vi "DIALOG_Method Selection.vi"(7 "Action":T6, 8 "Error In":errorcluster, 9 "User VI Ref":refnum<vi>, 10 "Affected Items":T4, 11 "Methods for Tree In":T5(array[cluster])=[{"Label"="Divider", "Tag"="0,6,MCListbox (strict),Divider,Divider", "Property Type"=enum."Divider", "Indent"=0, "Can Read?"=FALSE, "Can Write?"=FALSE, "Is Read?"=FALSE, "Is Write?"=FALSE, "Inactive Parent?"=FALSE, "Unwired?"=FALSE}, {"Label"="Class Operator", "Tag"="1,2,MCListbox (strict),6327405,Class Operator", "Property Type"=enum."Base", "Indent"=0, "Can Read?"=FALSE, "Can Write?"=FALSE, "Is Read?"=FALSE, "Is Write?"=FALSE, "Inactive Parent?"=TRUE, "Unwired?"=FALSE}, {"Label"="Call", "Tag"="1,2,MCListbox (strict),6327405,Class Operator:Call", "Property Type"=enum."Scripting", "Indent"=1, "Can Read?"=FALSE, "Can Write?"=FALSE, "Is Read?"=FALSE, "Is Write?"=FALSE, "Inactive Parent?"=FALSE, "Unwired?"=FALSE}, {"Label"="Traverse", "Tag"="2,2,MCListbox (strict),6327406,Class Operator:Traverse", "Property Type"=enum."Scripting", "Indent"=1, "Can Read?"=FALSE, "Can Write?"=FALSE, "Is Read?"=FALSE, "Is Write?"=FALSE, "Inactive Parent?"=FALSE, "Unwired?"=FALSE}, {"Label"="Delete", "Tag"="3,2,MCListbox (strict),6327400,Delete", "Property Type"=enum."Scripting", "Indent"=0, "Can Read?"=FALSE, "Can Write?"=FALSE, "Is Read?"=FALSE, "Is Write?"=FALSE, "Inactive Parent?"=FALSE, "Unwired?"=FALSE}, {"Label"="Get Property", "Tag"="4,3,MCListbox (strict),6327408,Get Property", "Property Type"=enum."Private", "Indent"=0, "Can Read?"=FALSE, "Can Write?"=FALSE, "Is Read?"=FALSE, "Is Write?"=FALSE, "Inactive Parent?"=FALSE, "Unwired?"=FALSE}, {"Label"="Get Property Call Data", "Tag"="5,3,MCListbox (strict),6327409,Get Property Call Data", "Property Type"=enum."Private", "Indent"=0, "Can Read?"=FALSE, "Can Write?"=FALSE, "Is Read?"=FALSE, "Is Write?"=FALSE, "Inactive Parent?"=FALSE, "Unwired?"=FALSE}, {"Label"="NI Security", "Tag"="6,3,MCListbox (strict),632740b,NI Security", "Property Type"=enum."Base", "Indent"=0, "Can Read?"=FALSE, "Can Write?"=FALSE, "Is Read?"=FALSE, "Is Write?"=FALSE, "Inactive Parent?"=TRUE, "Unwired?"=FALSE}, {"Label"="Get Access Control List", "Tag"="6,3,MCListbox (strict),632740b,NI Security:Get Access Control List", "Property Type"=enum."Private", "Indent"=1, "Can Read?"=FALSE, "Can Write?"=FALSE, "Is Read?"=FALSE, "Is Write?"=FALSE, "Inactive Parent?"=FALSE, "Unwired?"=FALSE}, {"Label"="Remove Access Control List", "Tag"="7,3,MCListbox (strict),632740c,NI Security:Remove Access Control List", "Property Type"=enum."Private", "Indent"=1, "Can Read?"=FALSE, "Can Write?"=FALSE, "Is Read?"=FALSE, "Is Write?"=FALSE, "Inactive Parent?"=FALSE, "Unwired?"=FALSE}, {"Label"="Set Access Control List", "Tag"="8,3,MCListbox (strict),632740a,NI Security:Set Access Control List", "Property Type"=enum."Private", "Indent"=1, "Can Read?"=FALSE, "Can Write?"=FALSE, "Is Read?"=FALSE, "Is Write?"=FALSE, "Inactive Parent?"=FALSE, "Unwired?"=FALSE}, {"Label"="Set HeapDocMod For Object", "Tag"="9,3,MCListbox (strict),632740d,Set HeapDocMod For Object", "Property Type"=enum."Private", "Indent"=0, "Can Read?"=FALSE, "Can Write?"=FALSE, "Is Read?"=FALSE, "Is Write?"=FALSE, "Inactive Parent?"=FALSE, "Unwired?"=FALSE}, {"Label"="Set Property", "Tag"="10,3,MCListbox (strict),6327407,Set Property", "Property Type"=enum."Private", "Indent"=0, "Can Read?"=FALSE, "Can Write?"=FALSE, "Is Read?"=FALSE, "Is Write?"=FALSE, "Inactive Parent?"=FALSE, "Unwired?"=FALSE}, {"Label"="Tag", "Tag"="11,2,MCListbox (strict),6327403,Tag", "Property Type"=enum."Base", "Indent"=0, "Can Read?"=FALSE, "Can Write?"=FALSE, "Is Read?"=FALSE, "Is Write?"=FALSE, "Inactive Parent?"=TRUE, "Unwired?"=FALSE}, {"Label"="Get Tag", "Tag"="11,2,MCListbox (strict),6327403,Tag:Get Tag", "Property Type"=enum."Scripting", "Indent"=1, "Can Read?"=FALSE, "Can Write?"=FALSE, "Is Read?"=FALSE, "Is Write?"=FALSE, "Inactive Parent?"=FALSE, "Unwired?"=FALSE}, {"Label"="Remove Tag", "Tag"="12,2,MCListbox (strict),6327402,Tag:Remove Tag", "Property Type"=enum."Scripting", "Indent"=1, "Can Read?"=FALSE, "Can Write?"=FALSE, "Is Read?"=FALSE, "Is Write?"=FALSE, "Inactive Parent?"=FALSE, "Unwired?"=FALSE}, {"Label"="Set Tag", "Tag"="13,2,MCListbox (strict),6327401,Tag:Set Tag", "Property Type"=enum."Scripting", "Indent"=1, "Can Read?"=FALSE, "Can Write?"=FALSE, "Is Read?"=FALSE, "Is Write?"=FALSE, "Inactive Parent?"=FALSE, "Unwired?"=FALSE}, {"Label"="Set Tag Persistence", "Tag"="14,2,MCListbox (strict),6327404,Tag:Set Tag Persistence", "Property Type"=enum."Scripting", "Indent"=1, "Can Read?"=FALSE, "Can Write?"=FALSE, "Is Read?"=FALSE, "Is Write?"=FALSE, "Inactive Parent?"=FALSE, "Unwired?"=FALSE}, {"Label"="Divider", "Tag"="15,6,MCListbox (strict),Divider,Divider", "Property Type"=enum."Divider", "Indent"=0, "Can Read?"=FALSE, "Can Write?"=FALSE, "Is Read?"=FALSE, "Is Write?"=FALSE, "Inactive Parent?"=FALSE, "Unwired?"=FALSE}, {"Label"="Get Help Info", "Tag"="16,2,MCListbox (strict),632a407,Get Help Info", "Property Type"=enum."Scripting", "Indent"=0, "Can Read?"=FALSE, "Can Write?"=FALSE, "Is Read?"=FALSE, "Is Write?"=FALSE, "Inactive Parent?"=FALSE, "Unwired?"=FALSE}, {"Label"="Invalidate", "Tag"="17,3,MCListbox (strict),632a405,Invalidate", "Property Type"=enum."Private", "Indent"=0, "Can Read?"=FALSE, "Can Write?"=FALSE, "Is Read?"=FALSE, "Is Write?"=FALSE, "Inactive Parent?"=FALSE, "Unwired?"=FALSE}, {"Label"="Launch Config Page", "Tag"="18,3,MCListbox (strict),632a404,Launch Config Page", "Property Type"=enum."Private", "Indent"=0, "Can Read?"=FALSE, "Can Write?"=FALSE, "Is Read?"=FALSE, "Is Write?"=FALSE, "Inactive Parent?"=FALSE, "Unwired?"=FALSE}, {"Label"="Move", "Tag"="19,2,MCListbox (strict),632a400,Move", "Property Type"=enum."Scripting", "Indent"=0, "Can Read?"=FALSE, "Can Write?"=FALSE, "Is Read?"=FALSE, "Is Write?"=FALSE, "Inactive Parent?"=FALSE, "Unwired?"=FALSE}, {"Label"="Object Highlight", "Tag"="20,1,MCListbox (strict),632a401,Object Highlight", "Property Type"=enum."Base", "Indent"=0, "Can Read?"=FALSE, "Can Write?"=FALSE, "Is Read?"=FALSE, "Is Write?"=FALSE, "Inactive Parent?"=FALSE, "Unwired?"=FALSE}, {"Label"="Replace", "Tag"="21,2,MCListbox (strict),632a402,Replace", "Property Type"=enum."Scripting", "Indent"=0, "Can Read?"=FALSE, "Can Write?"=FALSE, "Is Read?"=FALSE, "Is Write?"=FALSE, "Inactive Parent?"=FALSE, "Unwired?"=FALSE}, {"Label"="Replace No Attributes", "Tag"="22,2,MCListbox (strict),632a403,Replace No Attributes", "Property Type"=enum."Scripting", "Indent"=0, "Can Read?"=FALSE, "Can Write?"=FALSE, "Is Read?"=FALSE, "Is Write?"=FALSE, "Inactive Parent?"=FALSE, "Unwired?"=FALSE}, {"Label"="Replace Preferring Stub DDO OnFP", "Tag"="23,3,MCListbox (strict),632a406,Replace Preferring Stub DDO OnFP", "Property Type"=enum."Private", "Indent"=0, "Can Read?"=FALSE, "Can Write?"=FALSE, "Is Read?"=FALSE, "Is Write?"=FALSE, "Inactive Parent?"=FALSE, "Unwired?"=FALSE}, {"Label"="Divider", "Tag"="24,6,MCListbox (strict),Divider,Divider", "Property Type"=enum."Divider", "Indent"=0, "Can Read?"=FALSE, "Can Write?"=FALSE, "Is Read?"=FALSE, "Is Write?"=FALSE, "Inactive Parent?"=FALSE, "Unwired?"=FALSE}, {"Label"="Attach DataSocket", "Tag"="25,1,MCListbox (strict),6331c06,Attach DataSocket", "Property Type"=enum."Base", "Indent"=0, "Can Read?"=FALSE, "Can Write?"=FALSE, "Is Read?"=FALSE, "Is Write?"=FALSE, "Inactive Parent?"=FALSE, "Unwired?"=FALSE}, {"Label"="Copy Wizard Template", "Tag"="26,3,MCListbox (strict),6331c08,Copy Wizard Template", "Property Type"=enum."Private", "Indent"=0, "Can Read?"=FALSE, "Can Write?"=FALSE, "Is Read?"=FALSE, "Is Write?"=FALSE, "Inactive Parent?"=FALSE, "Unwired?"=FALSE}, {"Label"="Create", "Tag"="27,2,MCListbox (strict),6331c01,Create", "Property Type"=enum."Base", "Indent"=0, "Can Read?"=FALSE, "Can Write?"=FALSE, "Is Read?"=FALSE, "Is Write?"=FALSE, "Inactive Parent?"=TRUE, "Unwired?"=FALSE}, {"Label"="Control Reference", "Tag"="27,2,MCListbox (strict),6331c01,Create:Control Reference", "Property Type"=enum."Scripting", "Indent"=1, "Can Read?"=FALSE, "Can Write?"=FALSE, "Is Read?"=FALSE, "Is Write?"=FALSE, "Inactive Parent?"=FALSE, "Unwired?"=FALSE}, {"Label"="Invoke Node", "Tag"="28,2,MCListbox (strict),6331c04,Create:Invoke Node", "Property Type"=enum."Scripting", "Indent"=1, "Can Read?"=FALSE, "Can Write?"=FALSE, "Is Read?"=FALSE, "Is Write?"=FALSE, "Inactive Parent?"=FALSE, "Unwired?"=FALSE}, {"Label"="Local Variable", "Tag"="29,2,MCListbox (strict),6331c02,Create:Local Variable", "Property Type"=enum."Scripting", "Indent"=1, "Can Read?"=FALSE, "Can Write?"=FALSE, "Is Read?"=FALSE, "Is Write?"=FALSE, "Inactive Parent?"=FALSE, "Unwired?"=FALSE}, {"Label"="Property Node", "Tag"="30,2,MCListbox (strict),6331c03,Create:Property Node", "Property Type"=enum."Scripting", "Indent"=1, "Can Read?"=FALSE, "Can Write?"=FALSE, "Is Read?"=FALSE, "Is Write?"=FALSE, "Inactive Parent?"=FALSE, "Unwired?"=FALSE}, {"Label"="Data Binding", "Tag"="31,1,MCListbox (strict),6331c0f,Data Binding", "Property Type"=enum."Base", "Indent"=0, "Can Read?"=FALSE, "Can Write?"=FALSE, "Is Read?"=FALSE, "Is Write?"=FALSE, "Inactive Parent?"=TRUE, "Unwired?"=FALSE}, {"Label"="Bind To Network Path", "Tag"="31,1,MCListbox (strict),6331c0f,Data Binding:Bind To Network Path", "Property Type"=enum."Base", "Indent"=1, "Can Read?"=FALSE, "Can Write?"=FALSE, "Is Read?"=FALSE, "Is Write?"=FALSE, "Inactive Parent?"=FALSE, "Unwired?"=FALSE}, {"Label"="Bind To Network Variable", "Tag"="32,3,MCListbox (strict),6331c11,Data Binding:Bind To Network Variable", "Property Type"=enum."Private", "Indent"=1, "Can Read?"=FALSE, "Can Write?"=FALSE, "Is Read?"=FALSE, "Is Write?"=FALSE, "Inactive Parent?"=FALSE, "Unwired?"=FALSE}, {"Label"="Unbind", "Tag"="33,1,MCListbox (strict),6331c12,Data Binding:Unbind", "Property Type"=enum."Base", "Indent"=1, "Can Read?"=FALSE, "Can Write?"=FALSE, "Is Read?"=FALSE, "Is Write?"=FALSE, "Inactive Parent?"=FALSE, "Unwired?"=FALSE}, {"Label"="Data Operations", "Tag"="34,2,MCListbox (strict),6331c14,Data Operations", "Property Type"=enum."Base", "Indent"=0, "Can Read?"=FALSE, "Can Write?"=FALSE, "Is Read?"=FALSE, "Is Write?"=FALSE, "Inactive Parent?"=TRUE, "Unwired?"=FALSE}, {"Label"="Copy Data", "Tag"="34,2,MCListbox (strict),6331c14,Data Operations:Copy Data", "Property Type"=enum."Scripting", "Indent"=1, "Can Read?"=FALSE, "Can Write?"=FALSE, "Is Read?"=FALSE, "Is Write?"=FALSE, "Inactive Parent?"=FALSE, "Unwired?"=FALSE}, {"Label"="Paste Data", "Tag"="35,2,MCListbox (strict),6331c15,Data Operations:Paste Data", "Property Type"=enum."Scripting", "Indent"=1, "Can Read?"=FALSE, "Can Write?"=FALSE, "Is Read?"=FALSE, "Is Write?"=FALSE, "Inactive Parent?"=FALSE, "Unwired?"=FALSE}, {"Label"="Disconnect From Typedef", "Tag"="36,2,MCListbox (strict),6331c09,Disconnect From Typedef", "Property Type"=enum."Scripting", "Indent"=0, "Can Read?"=FALSE, "Can Write?"=FALSE, "Is Read?"=FALSE, "Is Write?"=FALSE, "Inactive Parent?"=FALSE, "Unwired?"=FALSE}, {"Label"="Fit Control To Pane", "Tag"="37,1,MCListbox (strict),6331c13,Fit Control To Pane", "Property Type"=enum."Base", "Indent"=0, "Can Read?"=FALSE, "Can Write?"=FALSE, "Is Read?"=FALSE, "Is Write?"=FALSE, "Inactive Parent?"=FALSE, "Unwired?"=FALSE}, {"Label"="Get Image", "Tag"="38,1,MCListbox (strict),6331c0c,Get Image", "Property Type"=enum."Base", "Indent"=0, "Can Read?"=FALSE, "Can Write?"=FALSE, "Is Read?"=FALSE, "Is Write?"=FALSE, "Inactive Parent?"=FALSE, "Unwired?"=FALSE}, {"Label"="Get Terminal Image", "Tag"="39,1,MCListbox (strict),6331c0d,Get Terminal Image", "Property Type"=enum."Base", "Indent"=0, "Can Read?"=FALSE, "Can Write?"=FALSE, "Is Read?"=FALSE, "Is Write?"=FALSE, "Inactive Parent?"=FALSE, "Unwired?"=FALSE}, {"Label"="Reinitialize To Default", "Tag"="40,1,MCListbox (strict),6331c00,Reinitialize To Default", "Property Type"=enum."Base", "Indent"=0, "Can Read?"=FALSE, "Can Write?"=FALSE, "Is Read?"=FALSE, "Is Write?"=FALSE, "Inactive Parent?"=FALSE, "Unwired?"=FALSE}, {"Label"="Remove DataSocket", "Tag"="41,1,MCListbox (strict),6331c07,Remove DataSocket", "Property Type"=enum."Base", "Indent"=0, "Can Read?"=FALSE, "Can Write?"=FALSE, "Is Read?"=FALSE, "Is Write?"=FALSE, "Inactive Parent?"=FALSE, "Unwired?"=FALSE}, {"Label"="Start Drag", "Tag"="42,1,MCListbox (strict),6331c0e,Start Drag", "Property Type"=enum."Base", "Indent"=0, "Can Read?"=FALSE, "Can Write?"=FALSE, "Is Read?"=FALSE, "Is Write?"=FALSE, "Inactive Parent?"=FALSE, "Unwired?"=FALSE}, {"Label"="Stub", "Tag"="43,3,MCListbox (strict),6331c16,Stub", "Property Type"=enum."Base", "Indent"=0, "Can Read?"=FALSE, "Can Write?"=FALSE, "Is Read?"=FALSE, "Is Write?"=FALSE, "Inactive Parent?"=TRUE, "Unwired?"=FALSE}, {"Label"="Convert To Stub", "Tag"="43,3,MCListbox (strict),6331c16,Stub:Convert To Stub", "Property Type"=enum."Private", "Indent"=1, "Can Read?"=FALSE, "Can Write?"=FALSE, "Is Read?"=FALSE, "Is Write?"=FALSE, "Inactive Parent?"=FALSE, "Unwired?"=FALSE}, {"Label"="Revert From Stub", "Tag"="44,3,MCListbox (strict),6331c17,Stub:Revert From Stub", "Property Type"=enum."Private", "Indent"=1, "Can Read?"=FALSE, "Can Write?"=FALSE, "Is Read?"=FALSE, "Is Write?"=FALSE, "Inactive Parent?"=FALSE, "Unwired?"=FALSE}, {"Label"="Update From Typedef", "Tag"="45,2,MCListbox (strict),6331c0a,Update From Typedef", "Property Type"=enum."Scripting", "Indent"=0, "Can Read?"=FALSE, "Can Write?"=FALSE, "Is Read?"=FALSE, "Is Write?"=FALSE, "Inactive Parent?"=FALSE, "Unwired?"=FALSE}, {"Label"="Divider", "Tag"="46,6,MCListbox (strict),Divider,Divider", "Property Type"=enum."Divider", "Indent"=0, "Can Read?"=FALSE, "Can Write?"=FALSE, "Is Read?"=FALSE, "Is Write?"=FALSE, "Inactive Parent?"=FALSE, "Unwired?"=FALSE}, {"Label"="Custom Item Symbols", "Tag"="47,1,MCListbox (strict),18d99403,Custom Item Symbols", "Property Type"=enum."Base", "Indent"=0, "Can Read?"=FALSE, "Can Write?"=FALSE, "Is Read?"=FALSE, "Is Write?"=FALSE, "Inactive Parent?"=TRUE, "Unwired?"=FALSE}, {"Label"="Get Symbol", "Tag"="47,1,MCListbox (strict),18d99403,Custom Item Symbols:Get Symbol", "Property Type"=enum."Base", "Indent"=1, "Can Read?"=FALSE, "Can Write?"=FALSE, "Is Read?"=FALSE, "Is Write?"=FALSE, "Inactive Parent?"=FALSE, "Unwired?"=FALSE}, {"Label"="Get Symbol Array", "Tag"="48,1,MCListbox (strict),18d99404,Custom Item Symbols:Get Symbol Array", "Property Type"=enum."Base", "Indent"=1, "Can Read?"=FALSE, "Can Write?"=FALSE, "Is Read?"=FALSE, "Is Write?"=FALSE, "Inactive Parent?"=FALSE, "Unwired?"=FALSE}, {"Label"="Revert All To Built In Symbols", "Tag"="49,1,MCListbox (strict),18d99408,Custom Item Symbols:Revert All To Built In Symbols", "Property Type"=enum."Base", "Indent"=1, "Can Read?"=FALSE, "Can Write?"=FALSE, "Is Read?"=FALSE, "Is Write?"=FALSE, "Inactive Parent?"=FALSE, "Unwired?"=FALSE}, {"Label"="Revert To Built In Symbol", "Tag"="50,1,MCListbox (strict),18d99407,Custom Item Symbols:Revert To Built In Symbol", "Property Type"=enum."Base", "Indent"=1, "Can Read?"=FALSE, "Can Write?"=FALSE, "Is Read?"=FALSE, "Is Write?"=FALSE, "Inactive Parent?"=FALSE, "Unwired?"=FALSE}, {"Label"="Set To Custom Symbol", "Tag"="51,1,MCListbox (strict),18d99405,Custom Item Symbols:Set To Custom Symbol", "Property Type"=enum."Base", "Indent"=1, "Can Read?"=FALSE, "Can Write?"=FALSE, "Is Read?"=FALSE, "Is Write?"=FALSE, "Inactive Parent?"=FALSE, "Unwired?"=FALSE}, {"Label"="Set To Custom Symbol Array", "Tag"="52,1,MCListbox (strict),18d99406,Custom Item Symbols:Set To Custom Symbol Array", "Property Type"=enum."Base", "Indent"=1, "Can Read?"=FALSE, "Can Write?"=FALSE, "Is Read?"=FALSE, "Is Write?"=FALSE, "Inactive Parent?"=FALSE, "Unwired?"=FALSE}, {"Label"="Get Clicked Column Header", "Tag"="53,1,MCListbox (strict),18d99401,Get Clicked Column Header", "Property Type"=enum."Base", "Indent"=0, "Can Read?"=FALSE, "Can Write?"=FALSE, "Is Read?"=FALSE, "Is Write?"=FALSE, "Inactive Parent?"=FALSE, "Unwired?"=FALSE}, {"Label"="Get Double-Clicked Row", "Tag"="54,1,MCListbox (strict),18d99400,Get Double-Clicked Row", "Property Type"=enum."Base", "Indent"=0, "Can Read?"=FALSE, "Can Write?"=FALSE, "Is Read?"=FALSE, "Is Write?"=FALSE, "Inactive Parent?"=FALSE, "Unwired?"=FALSE}, {"Label"="Point to Row Column", "Tag"="55,1,MCListbox (strict),18d99402,Point to Row Column", "Property Type"=enum."Base", "Indent"=0, "Can Read?"=FALSE, "Can Write?"=FALSE, "Is Read?"=FALSE, "Is Write?"=FALSE, "Inactive Parent?"=FALSE, "Unwired?"=FALSE}]) -> (0 "Error Out":errorcluster, 2 "Placement Out":enum32{"Choice 1", "Choice 2"}(radio), 3 "Method Array Out":T3(array[cluster]))   [LabVIEW 2023]
doc: "Dialog to select items from the input cluster ref. \n\nFilter narrows list of items.\nDown key puts focus on tree and selects first item.\nUp and Down keps navigate tree.\nMultiple items can be selected.\n\nIn case of action \"Delete\" (\"Remove elements(s)...\" selected), list will show all elements currently displayed, else it will show all elements availabel to undle or unbundle.\n\nOutput is a list of the selected item tags."
uses:
  controls/action enum.ctl
  top/BundleMagic.ctl
  controls/Done Button.ctl
panel:
  in  "Filter":string
  in  "Tree":string[](tree)
  in  "Placement":enum32{"Choice 1", "Choice 2"}(radio)
  in  "Property Display":T1
  in  "Done":T2
  in  "Show radio":bool
  # "Debug"
  # "use same format as prop arry, but only tag matters here"
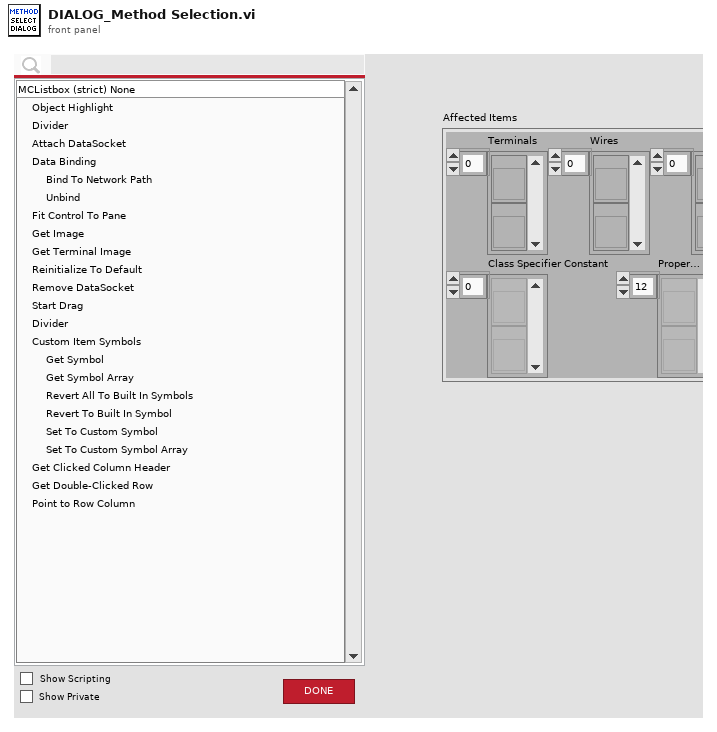
[diagram p1: front panel]
types:
  T1 = cluster{"Show Scripting":bool, "Show Private":bool}
  T2 = typedef "Done Button.ctl" = bool
  T3 = cluster{"Tag":string, "Read":bool, "Write":bool, "New":bool}[]
  T4 = typedef "BundleMagic.ctl" = cluster{"Terminals":refnum<vi>[], "Wires":refnum<vi>[], "Named Bundler":refnum<vi>[], "Named Unbundler":refnum<vi>[], "In Place Cluster Node":refnum<vi>[], "Class Specifier Constant":refnum<vi>[], "Property Node":refnum<vi>[], "Invoke Node":refnum<vi>[], "Refnum Control":refnum<vi>[]}
  T5 = cluster{"Label":string, "Tag":string, "Property Type":enum16{"Unknown", "Base", "Scripting", "Private", "Deprecated", "None", "Divider"}, "Indent":u16, "Can Read?":bool, "Can Write?":bool, "Is Read?":bool, "Is Write?":bool, "Inactive Parent?":bool, "Unwired?":bool}[]
  T6 = typedef "action enum.ctl" = enum16{"[NONE]", "Wire Bundle", "Wire Unbundle", "Terminal Unbundle", "Terminal Bundle", "Bundler Move Up", "Bundler Move Down", "Bundler Insert", "Bundler Remove", "Bundler Remove Unwired", "Bundler Rearrange", "In Place Insert", "In Place Remove", "In Place Remove Unwired", "In Place Rearrange", "Wire Properties", "Wire Method", "Terminal Properties", "Terminal Method", "Property Move Up", "Property Move Down", "Properties Insert", "Properties Remove", "Properties Remove Unwired", "Properties Rearrange", "Method Change", "Class For Constant", "Class For Control", "Class For Node", "Class Name to Clipboard"}
  T7 = typedef "eventvkey.ctl" = enum16{"ASCII", "Enter", "Return", "Shift", "Ctrl", "Alt", "Cmd", "Opt", "Caps", "NumLock", "Clear", "Break", "Up", "Down", "Left", "Right", "Insert", "Delete", "Home", "End", "PageUp", "PageDown", "Escape", "Help", "Pause", "ScrollLock", "F1", "F2", "F3", "F4", "F5", "F6", "F7", "F8", "F9", "F10", "F11", "F12", "F13", "F14", "F15", "F16", "F17", "F18", "F19", "F20", "F21", "F22", "F23", "F24", "Play", "VolumeUp", "VolumeDown", "Mute", "Two Byte Char"}
  T8 = cluster{"Tag":string, "Read":bool, "Write":bool, "New":bool}
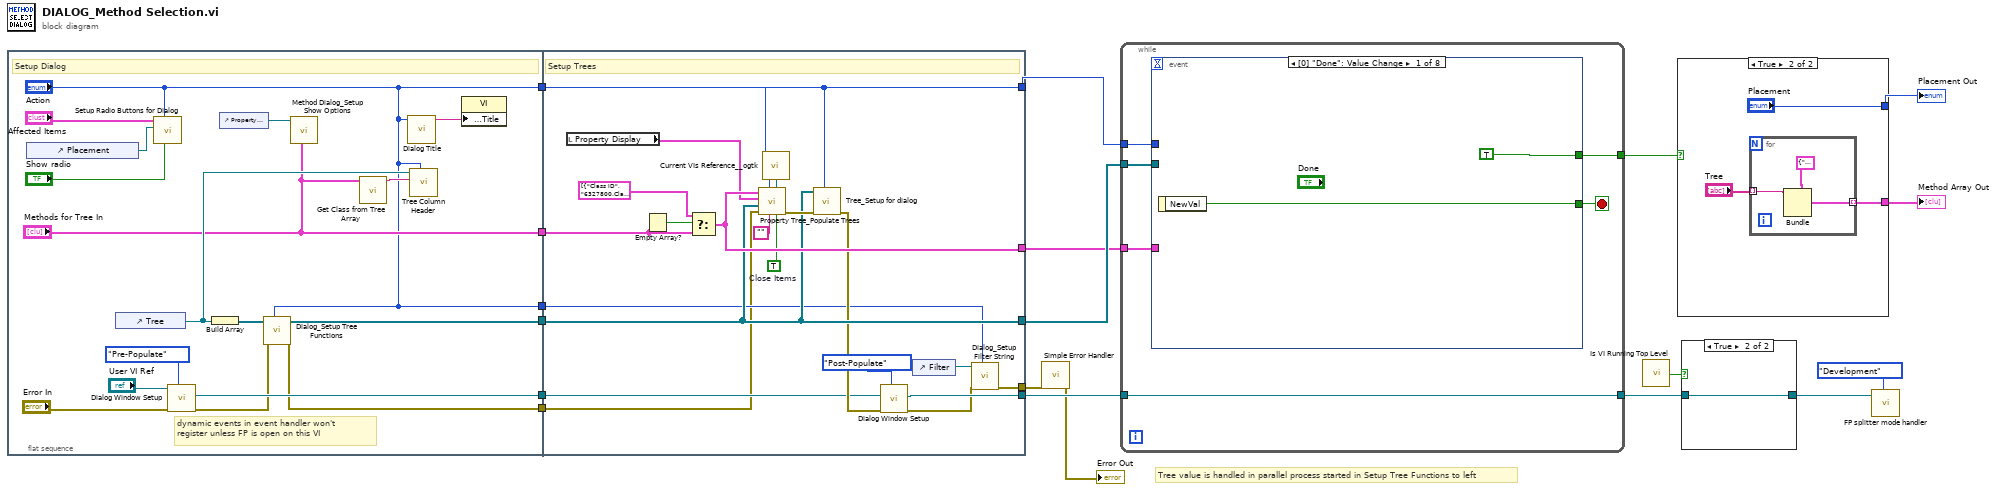
[diagram p0: block diagram]
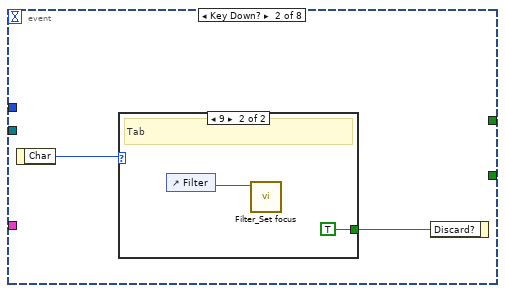
[diagram p2: hidden frame]
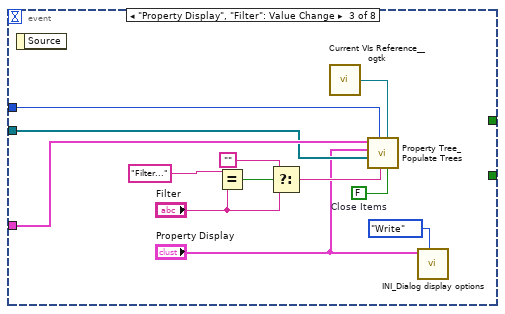
[diagram p4: hidden frame]
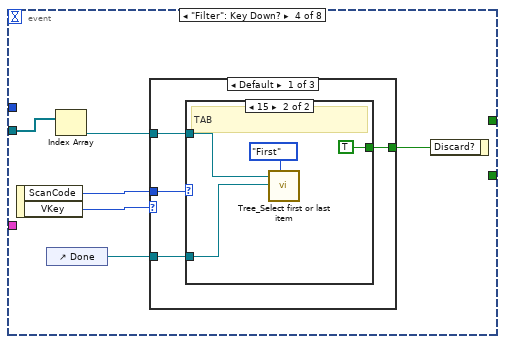
[diagram p5: hidden frame]
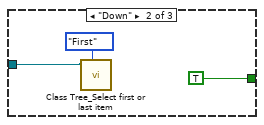
[diagram p7: hidden frame]
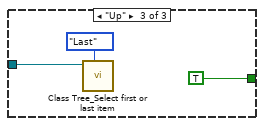
[diagram p8: hidden frame]
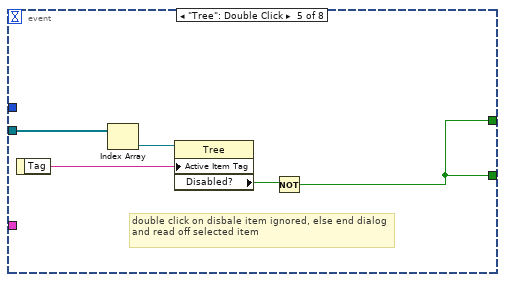
[diagram p9: hidden frame]
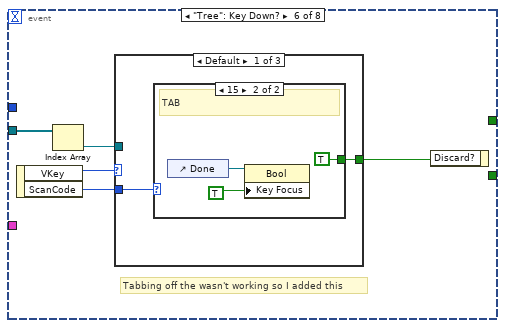
[diagram p10: hidden frame]
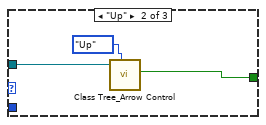
[diagram p12: hidden frame]
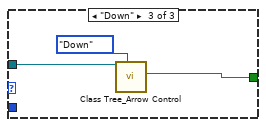
[diagram p13: hidden frame]
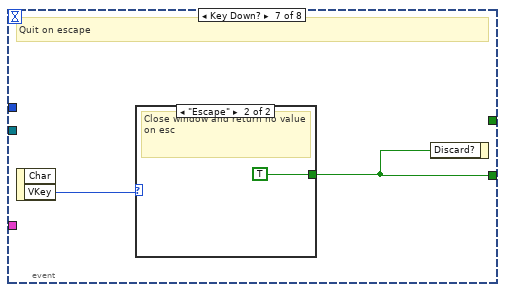
[diagram p14: hidden frame]
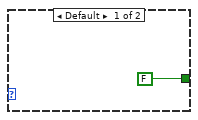
[diagram p15: hidden frame]
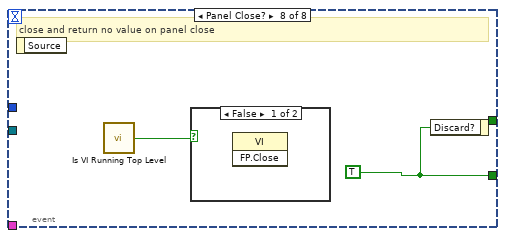
[diagram p16: hidden frame]
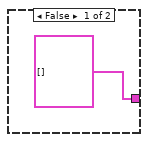
[diagram p18: hidden frame]
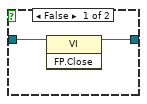
[diagram p19: hidden frame]
diagram:
  # "Tree value is handled in parallel process started in Setup Tree Functions to left"
  n1 = flat-sequence {
    tunnel: [w33] -> w12
    tunnel: [w31] -> w11
    tunnel: ["Action"] -> w10
    tunnel: ["Methods for Tree In"] -> w6
    tunnel: ["Action"] -> w4
    tunnel: [w21] -> w3
    tunnel: [w51] -> w13
    tunnel: [w43] -> w17
    tunnel: w12 -> [w44]
    tunnel: w11 -> [w51]
    tunnel: [w53] -> w7
    tunnel: w10 -> [w52]
    tunnel: [w52] -> w9
    tunnel: w6 -> [w47]
    tunnel: w4 -> [w39]
    tunnel: w3 -> [w38]
    tunnel: [w37] -> w2
    frame #0 {
      # "dynamic events in event handler won't register unless FP is open on this VI"
      # "Setup Dialog"
      n2 = control-ref of="Placement"() -> (w29:refnum<vi>)
      n3 = control-ref of="Tree"() -> (w25:refnum<vi>)
      n4 = call "Setup Radio Buttons for Dialog.vi"("Show Radio"="Show radio", "Action"="Action", "Action Choice Ref"=w29, "Affected Items"="Affected Items") -> ()  [unwired: 8 in]
      n5 = call "Dialog Window Setup.vi"("Action"=enum16{"Pre-Populate", "Post-Populate"}."Pre-Populate", "error in"="Error In", "Align-to Window Ref"="User VI Ref") -> ("error out"=w32:errorcluster, "Dialog VI Ref Out"=w33:refnum<vi>)  [unwired: 7 in]
      n6 = Build Array(w25) -> (w30:refnum<vi>[])
      n7 = control-ref of="Property Display"() -> (w28:refnum<vi>)
      n8 = call "Dialog_Setup Tree Functions.vi"("Action"="Action", "error in"=w32, "Tree Ref Array In"=w30) -> ("error out"=w21:errorcluster, "Tree Ref Array Out"=w31:refnum<vi>[])  [unwired: 7 in]
      n9 = call "Method Dialog_Setup Show Options.vi"("Properties for Tree In"="Methods for Tree In", "Cluster in"=w28) -> ()  [unwired: 10 in]
      n10 = call "Get Class from Tree Array.vi"("Methods for Tree In"="Methods for Tree In") -> ("Class"=w24:string)  [unwired: 10 in]
      n11 = call "Dialog Title.vi"("Action"="Action") -> ("Window Title"=w27:string)  [unwired: 10 in]
      n12 = call "Tree Column Header.vi"("Action"="Action", "Class Name"=w24, "Tree Ref"=w25) -> ()  [unwired: 8 in, 1 out]
      n13 = property class="VI"("Front Panel.Title"=w27) -> ()  [unwired: 2 in, 2 out]
    }
    frame #1 {
      w46 = TRUE  # Close Items
      # "Setup Trees"
      n14 = local read "Property Display"() -> (w50:T1)
      n15 = Empty Array?(array=w47) -> (empty?=w56:bool)
      n16 = Select(t=T5 [{"Label"="Class ID", "Tag"="6327800.Class ID", "Property Type"=enum."Base", "Indent"=0, "Can Read?"=TRUE, "Can Write?"=FALSE, "Is Read?"=FALSE, "Is Write?"=FALSE, "Inactive Parent?"=FALSE, "Unwired?"=FALSE}, {"Label"="Class Name", "Tag"="6327803.Class Name", "Property Type"=enum."Base", "Indent"=0, "Can Read?"=TRUE, "Can Write?"=FALSE, "Is Read?"=FALSE, "Is Write?"=FALSE, "Inactive Parent?"=FALSE, "Unwired?"=FALSE}, {"Label"="Is On Block Diagram?", "Tag"="6327805.Is On Block Diagram?", "Property Type"=enum."Scripting", "Indent"=0, "Can Read?"=TRUE, "Can Write?"=FALSE, "Is Read?"=FALSE, "Is Write?"=FALSE, "Inactive Parent?"=FALSE, "Unwired?"=FALSE}, {"Label"="Modified", "Tag"="6327804.Modified", "Property Type"=enum."Private", "Indent"=0, "Can Read?"=TRUE, "Can Write?"=FALSE, "Is Read?"=FALSE, "Is Write?"=FALSE, "Inactive Parent?"=FALSE, "Unwired?"=FALSE}, {"Label"="Owner", "Tag"="6327806.Owner", "Property Type"=enum."Base", "Indent"=0, "Can Read?"=TRUE, "Can Write?"=FALSE, "Is Read?"=FALSE, "Is Write?"=FALSE, "Inactive Parent?"=FALSE, "Unwired?"=FALSE}, {"Label"="Owning VI", "Tag"="6327802.Owning VI", "Property Type"=enum."Base", "Indent"=0, "Can Read?"=TRUE, "Can Write?"=FALSE, "Is Read?"=FALSE, "Is Write?"=FALSE, "Inactive Parent?"=FALSE, "Unwired?"=FALSE}, {"Label"="Basic Object Flags", "Tag"="632a80c.Basic Object Flags", "Property Type"=enum."Private", "Indent"=0, "Can Read?"=TRUE, "Can Write?"=TRUE, "Is Read?"=FALSE, "Is Write?"=FALSE, "Inactive Parent?"=FALSE, "Unwired?"=FALSE}, {"Label"="Bounds", "Tag"="632a803.Bounds", "Property Type"=enum."Base", "Indent"=0, "Can Read?"=TRUE, "Can Write?"=FALSE, "Is Read?"=FALSE, "Is Write?"=FALSE, "Inactive Parent?"=FALSE, "Unwired?"=FALSE}, {"Label"="Area Height", "Tag"="632a805.Bounds:Area Height", "Property Type"=enum."Base", "Indent"=1, "Can Read?"=TRUE, "Can Write?"=FALSE, "Is Read?"=FALSE, "Is Write?"=FALSE, "Inactive Parent?"=FALSE, "Unwired?"=FALSE}, {"Label"="Area Width", "Tag"="632a804.Bounds:Area Width", "Property Type"=enum."Base", "Indent"=1, "Can Read?"=TRUE, "Can Write?"=FALSE, "Is Read?"=FALSE, "Is Write?"=FALSE, "Inactive Parent?"=FALSE, "Unwired?"=FALSE}, {"Label"="Dependencies", "Tag"="Dependencies", "Property Type"=enum."Scripting", "Indent"=0, "Can Read?"=FALSE, "Can Write?"=FALSE, "Is Read?"=FALSE, "Is Write?"=FALSE, "Inactive Parent?"=TRUE, "Unwired?"=FALSE}, {"Label"="Found Dependency Names", "Tag"="632a817.Dependencies:Found Dependency Names", "Property Type"=enum."Scripting", "Indent"=1, "Can Read?"=TRUE, "Can Write?"=FALSE, "Is Read?"=FALSE, "Is Write?"=FALSE, "Inactive Parent?"=FALSE, "Unwired?"=FALSE}, {"Label"="Found Dependency Paths", "Tag"="632a816.Dependencies:Found Dependency Paths", "Property Type"=enum."Scripting", "Indent"=1, "Can Read?"=TRUE, "Can Write?"=FALSE, "Is Read?"=FALSE, "Is Write?"=FALSE, "Inactive Parent?"=FALSE, "Unwired?"=FALSE}, {"Label"="Missing Dependency Names", "Tag"="632a815.Dependencies:Missing Dependency Names", "Property Type"=enum."Scripting", "Indent"=1, "Can Read?"=TRUE, "Can Write?"=FALSE, "Is Read?"=FALSE, "Is Write?"=FALSE, "Inactive Parent?"=FALSE, "Unwired?"=FALSE}, {"Label"="Missing Dependency Paths", "Tag"="632a814.Dependencies:Missing Dependency Paths", "Property Type"=enum."Scripting", "Indent"=1, "Can Read?"=TRUE, "Can Write?"=FALSE, "Is Read?"=FALSE, "Is Write?"=FALSE, "Inactive Parent?"=FALSE, "Unwired?"=FALSE}, {"Label"="Group Member Refs[]", "Tag"="632a808.Group Member Refs[]", "Property Type"=enum."Private", "Indent"=0, "Can Read?"=TRUE, "Can Write?"=FALSE, "Is Read?"=FALSE, "Is Write?"=FALSE, "Inactive Parent?"=FALSE, "Unwired?"=FALSE}, {"Label"="Grouped", "Tag"="632a806.Grouped", "Property Type"=enum."Private", "Indent"=0, "Can Read?"=TRUE, "Can Write?"=FALSE, "Is Read?"=FALSE, "Is Write?"=FALSE, "Inactive Parent?"=FALSE, "Unwired?"=FALSE}, {"Label"="Is Wizard Locked", "Tag"="632a80d.Is Wizard Locked", "Property Type"=enum."Private", "Indent"=0, "Can Read?"=TRUE, "Can Write?"=FALSE, "Is Read?"=FALSE, "Is Write?"=FALSE, "Inactive Parent?"=FALSE, "Unwired?"=FALSE}, {"Label"="Locked", "Tag"="632a807.Locked", "Property Type"=enum."Private", "Indent"=0, "Can Read?"=TRUE, "Can Write?"=FALSE, "Is Read?"=FALSE, "Is Write?"=FALSE, "Inactive Parent?"=FALSE, "Unwired?"=FALSE}, {"Label"="Master Bounds Rect", "Tag"="632a80b.Master Bounds Rect", "Property Type"=enum."Scripting", "Indent"=0, "Can Read?"=TRUE, "Can Write?"=FALSE, "Is Read?"=FALSE, "Is Write?"=FALSE, "Inactive Parent?"=FALSE, "Unwired?"=FALSE}, {"Label"="Position", "Tag"="632a800.Position", "Property Type"=enum."Base", "Indent"=0, "Can Read?"=TRUE, "Can Write?"=TRUE, "Is Read?"=FALSE, "Is Write?"=FALSE, "Inactive Parent?"=FALSE, "Unwired?"=FALSE}, {"Label"="Left", "Tag"="632a801.Position:Left", "Property Type"=enum."Base", "Indent"=1, "Can Read?"=TRUE, "Can Write?"=TRUE, "Is Read?"=FALSE, "Is Write?"=FALSE, "Inactive Parent?"=FALSE, "Unwired?"=FALSE}, {"Label"="Top", "Tag"="632a802.Position:Top", "Property Type"=enum."Base", "Indent"=1, "Can Read?"=TRUE, "Can Write?"=TRUE, "Is Read?"=FALSE, "Is Write?"=FALSE, "Inactive Parent?"=FALSE, "Unwired?"=FALSE}, {"Label"="Resize Info", "Tag"="Resize Info", "Property Type"=enum."Private", "Indent"=0, "Can Read?"=FALSE, "Can Write?"=FALSE, "Is Read?"=FALSE, "Is Write?"=FALSE, "Inactive Parent?"=TRUE, "Unwired?"=FALSE}, {"Label"="Can Resize Horizontally", "Tag"="632a80f.Resize Info:Can Resize Horizontally", "Property Type"=enum."Private", "Indent"=1, "Can Read?"=TRUE, "Can Write?"=FALSE, "Is Read?"=FALSE, "Is Write?"=FALSE, "Inactive Parent?"=FALSE, "Unwired?"=FALSE}, {"Label"="Can Resize Vertically", "Tag"="632a810.Resize Info:Can Resize Vertically", "Property Type"=enum."Private", "Indent"=1, "Can Read?"=TRUE, "Can Write?"=FALSE, "Is Read?"=FALSE, "Is Write?"=FALSE, "Inactive Parent?"=FALSE, "Unwired?"=FALSE}, {"Label"="Include In Resize", "Tag"="632a812.Resize Info:Include In Resize", "Property Type"=enum."Private", "Indent"=1, "Can Read?"=TRUE, "Can Write?"=FALSE, "Is Read?"=FALSE, "Is Write?"=FALSE, "Inactive Parent?"=FALSE, "Unwired?"=FALSE}, {"Label"="Name in Resize Dialog", "Tag"="632a811.Resize Info:Name in Resize Dialog", "Property Type"=enum."Private", "Indent"=1, "Can Read?"=TRUE, "Can Write?"=FALSE, "Is Read?"=FALSE, "Is Write?"=FALSE, "Inactive Parent?"=FALSE, "Unwired?"=FALSE}, {"Label"="Selected", "Tag"="632a809.Selected", "Property Type"=enum."Scripting", "Indent"=0, "Can Read?"=TRUE, "Can Write?"=TRUE, "Is Read?"=FALSE, "Is Write?"=FALSE, "Inactive Parent?"=FALSE, "Unwired?"=FALSE}, {"Label"="Total Bounds Rect", "Tag"="632a80a.Total Bounds Rect", "Property Type"=enum."Scripting", "Indent"=0, "Can Read?"=TRUE, "Can Write?"=FALSE, "Is Read?"=FALSE, "Is Write?"=FALSE, "Inactive Parent?"=FALSE, "Unwired?"=FALSE}, {"Label"="UID", "Tag"="632a813.UID", "Property Type"=enum."Scripting", "Indent"=0, "Can Read?"=TRUE, "Can Write?"=FALSE, "Is Read?"=FALSE, "Is Write?"=FALSE, "Inactive Parent?"=FALSE, "Unwired?"=FALSE}, {"Label"="Auto-Update From Typedef", "Tag"="633201c.Auto-Update From Typedef", "Property Type"=enum."Scripting", "Indent"=0, "Can Read?"=TRUE, "Can Write?"=TRUE, "Is Read?"=FALSE, "Is Write?"=FALSE, "Inactive Parent?"=FALSE, "Unwired?"=FALSE}, {"Label"="Bit Accurate Data Size", "Tag"="633201d.Bit Accurate Data Size", "Property Type"=enum."Private", "Indent"=0, "Can Read?"=TRUE, "Can Write?"=FALSE, "Is Read?"=FALSE, "Is Write?"=FALSE, "Inactive Parent?"=FALSE, "Unwired?"=FALSE}, {"Label"="Blinking", "Tag"="6332003.Blinking", "Property Type"=enum."Base", "Indent"=0, "Can Read?"=TRUE, "Can Write?"=TRUE, "Is Read?"=FALSE, "Is Write?"=FALSE, "Inactive Parent?"=FALSE, "Unwired?"=FALSE}, {"Label"="Built-In Mouse Wheel Support", "Tag"="633203f.Built-In Mouse Wheel Support", "Property Type"=enum."Base", "Indent"=0, "Can Read?"=TRUE, "Can Write?"=TRUE, "Is Read?"=FALSE, "Is Write?"=FALSE, "Inactive Parent?"=FALSE, "Unwired?"=FALSE}, {"Label"="C Type", "Tag"="6332026.C Type", "Property Type"=enum."Private", "Indent"=0, "Can Read?"=TRUE, "Can Write?"=FALSE, "Is Read?"=FALSE, "Is Write?"=FALSE, "Inactive Parent?"=FALSE, "Unwired?"=FALSE}, {"Label"="Caption", "Tag"="6332004.Caption", "Property Type"=enum."Base", "Indent"=0, "Can Read?"=TRUE, "Can Write?"=FALSE, "Is Read?"=FALSE, "Is Write?"=FALSE, "Inactive Parent?"=FALSE, "Unwired?"=FALSE}, {"Label"="Control Index", "Tag"="6332040.Control Index", "Property Type"=enum."Base", "Indent"=0, "Can Read?"=TRUE, "Can Write?"=FALSE, "Is Read?"=FALSE, "Is Write?"=FALSE, "Inactive Parent?"=FALSE, "Unwired?"=FALSE}, {"Label"="Control Reference Nodes[]", "Tag"="6332009.Control Reference Nodes[]", "Property Type"=enum."Scripting", "Indent"=0, "Can Read?"=TRUE, "Can Write?"=FALSE, "Is Read?"=FALSE, "Is Write?"=FALSE, "Inactive Parent?"=FALSE, "Unwired?"=FALSE}, {"Label"="Data Binding", "Tag"="Data Binding", "Property Type"=enum."Base", "Indent"=0, "Can Read?"=FALSE, "Can Write?"=FALSE, "Is Read?"=FALSE, "Is Write?"=FALSE, "Inactive Parent?"=TRUE, "Unwired?"=FALSE}, {"Label"="Binding Type", "Tag"="633202d.Data Binding:Binding Type", "Property Type"=enum."Base", "Indent"=1, "Can Read?"=TRUE, "Can Write?"=FALSE, "Is Read?"=FALSE, "Is Write?"=FALSE, "Inactive Parent?"=FALSE, "Unwired?"=FALSE}, {"Label"="Blink On Alarm", "Tag"="633202e.Data Binding:Blink On Alarm", "Property Type"=enum."Private", "Indent"=1, "Can Read?"=TRUE, "Can Write?"=TRUE, "Is Read?"=FALSE, "Is Write?"=FALSE, "Inactive Parent?"=FALSE, "Unwired?"=FALSE}, {"Label"="LED Visible", "Tag"="633202b.Data Binding:LED Visible", "Property Type"=enum."Base", "Indent"=1, "Can Read?"=TRUE, "Can Write?"=TRUE, "Is Read?"=FALSE, "Is Write?"=FALSE, "Inactive Parent?"=FALSE, "Unwired?"=FALSE}, {"Label"="Mode", "Tag"="6332029.Data Binding:Mode", "Property Type"=enum."Base", "Indent"=1, "Can Read?"=TRUE, "Can Write?"=TRUE, "Is Read?"=FALSE, "Is Write?"=FALSE, "Inactive Parent?"=FALSE, "Unwired?"=FALSE}, {"Label"="Path", "Tag"="6332028.Data Binding:Path", "Property Type"=enum."Base", "Indent"=1, "Can Read?"=TRUE, "Can Write?"=TRUE, "Is Read?"=FALSE, "Is Write?"=FALSE, "Inactive Parent?"=FALSE, "Unwired?"=FALSE}, {"Label"="Persist ID", "Tag"="633202c.Data Binding:Persist ID", "Property Type"=enum."Private", "Indent"=1, "Can Read?"=TRUE, "Can Write?"=FALSE, "Is Read?"=FALSE, "Is Write?"=FALSE, "Inactive Parent?"=FALSE, "Unwired?"=FALSE}, {"Label"="Status", "Tag"="633202a.Data Binding:Status", "Property Type"=enum."Base", "Indent"=1, "Can Read?"=TRUE, "Can Write?"=FALSE, "Is Read?"=FALSE, "Is Write?"=FALSE, "Inactive Parent?"=FALSE, "Unwired?"=FALSE}, {"Label"="DataSocket", "Tag"="DataSocket", "Property Type"=enum."Base", "Indent"=0, "Can Read?"=FALSE, "Can Write?"=FALSE, "Is Read?"=FALSE, "Is Write?"=FALSE, "Inactive Parent?"=TRUE, "Unwired?"=FALSE}, {"Label"="Enabled", "Tag"="6332017.DataSocket:Enabled", "Property Type"=enum."Base", "Indent"=1, "Can Read?"=TRUE, "Can Write?"=TRUE, "Is Read?"=FALSE, "Is Write?"=FALSE, "Inactive Parent?"=FALSE, "Unwired?"=FALSE}, {"Label"="LED Visible", "Tag"="633201e.DataSocket:LED Visible", "Property Type"=enum."Base", "Indent"=1, "Can Read?"=TRUE, "Can Write?"=TRUE, "Is Read?"=FALSE, "Is Write?"=FALSE, "Inactive Parent?"=FALSE, "Unwired?"=FALSE}, {"Label"="Mode", "Tag"="6332016.DataSocket:Mode", "Property Type"=enum."Base", "Indent"=1, "Can Read?"=TRUE, "Can Write?"=TRUE, "Is Read?"=FALSE, "Is Write?"=FALSE, "Inactive Parent?"=FALSE, "Unwired?"=FALSE}, {"Label"="Status", "Tag"="6332018.DataSocket:Status", "Property Type"=enum."Base", "Indent"=1, "Can Read?"=TRUE, "Can Write?"=FALSE, "Is Read?"=FALSE, "Is Write?"=FALSE, "Inactive Parent?"=FALSE, "Unwired?"=FALSE}, {"Label"="URL", "Tag"="6332015.DataSocket:URL", "Property Type"=enum."Base", "Indent"=1, "Can Read?"=TRUE, "Can Write?"=TRUE, "Is Read?"=FALSE, "Is Write?"=FALSE, "Inactive Parent?"=FALSE, "Unwired?"=FALSE}, {"Label"="", "Tag"="", "Property Type"=enum."Base", "Indent"=0, "Can Read?"=FALSE, "Can Write?"=FALSE, "Is Read?"=FALSE, "Is Write?"=FALSE, "Inactive Parent?"=FALSE, "Unwired?"=FALSE}, {"Label"="Default Value (Undoable)", "Tag"="6332043.Default Value (Undoable)", "Property Type"=enum."Scripting", "Indent"=0, "Can Read?"=FALSE, "Can Write?"=TRUE, "Is Read?"=FALSE, "Is Write?"=FALSE, "Inactive Parent?"=FALSE, "Unwired?"=FALSE}, {"Label"="Description", "Tag"="633200f.Description", "Property Type"=enum."Base", "Indent"=0, "Can Read?"=TRUE, "Can Write?"=TRUE, "Is Read?"=FALSE, "Is Write?"=FALSE, "Inactive Parent?"=FALSE, "Unwired?"=FALSE}, {"Label"="Disabled", "Tag"="633203d.Disabled", "Property Type"=enum."Base", "Indent"=0, "Can Read?"=TRUE, "Can Write?"=TRUE, "Is Read?"=FALSE, "Is Write?"=FALSE, "Inactive Parent?"=FALSE, "Unwired?"=FALSE}, {"Label"="Focus Key Binding", "Tag"="6332010.Focus Key Binding", "Property Type"=enum."Base", "Indent"=0, "Can Read?"=TRUE, "Can Write?"=TRUE, "Is Read?"=FALSE, "Is Write?"=FALSE, "Inactive Parent?"=FALSE, "Unwired?"=FALSE}, {"Label"="Genericity", "Tag"="633203c.Genericity", "Property Type"=enum."Private", "Indent"=0, "Can Read?"=TRUE, "Can Write?"=TRUE, "Is Read?"=FALSE, "Is Write?"=FALSE, "Inactive Parent?"=FALSE, "Unwired?"=FALSE}, {"Label"="Grow Info", "Tag"="633202f.Grow Info", "Property Type"=enum."Scripting", "Indent"=0, "Can Read?"=TRUE, "Can Write?"=FALSE, "Is Read?"=FALSE, "Is Write?"=FALSE, "Inactive Parent?"=FALSE, "Unwired?"=FALSE}, {"Label"="Can Grow Horizontally", "Tag"="6332030.Grow Info:Can Grow Horizontally", "Property Type"=enum."Scripting", "Indent"=1, "Can Read?"=TRUE, "Can Write?"=FALSE, "Is Read?"=FALSE, "Is Write?"=FALSE, "Inactive Parent?"=FALSE, "Unwired?"=FALSE}, {"Label"="Can Grow Vertically", "Tag"="6332031.Grow Info:Can Grow Vertically", "Property Type"=enum."Scripting", "Indent"=1, "Can Read?"=TRUE, "Can Write?"=FALSE, "Is Read?"=FALSE, "Is Write?"=FALSE, "Inactive Parent?"=FALSE, "Unwired?"=FALSE}, {"Label"="Max Horizontally", "Tag"="6332034.Grow Info:Max Horizontally", "Property Type"=enum."Scripting", "Indent"=1, "Can Read?"=TRUE, "Can Write?"=FALSE, "Is Read?"=FALSE, "Is Write?"=FALSE, "Inactive Parent?"=FALSE, "Unwired?"=FALSE}, {"Label"="Max Vertically", "Tag"="6332035.Grow Info:Max Vertically", "Property Type"=enum."Scripting", "Indent"=1, "Can Read?"=TRUE, "Can Write?"=FALSE, "Is Read?"=FALSE, "Is Write?"=FALSE, "Inactive Parent?"=FALSE, "Unwired?"=FALSE}, {"Label"="Min Horizontally", "Tag"="6332032.Grow Info:Min Horizontally", "Property Type"=enum."Scripting", "Indent"=1, "Can Read?"=TRUE, "Can Write?"=FALSE, "Is Read?"=FALSE, "Is Write?"=FALSE, "Inactive Parent?"=FALSE, "Unwired?"=FALSE}, {"Label"="Min Vertically", "Tag"="6332033.Grow Info:Min Vertically", "Property Type"=enum."Scripting", "Indent"=1, "Can Read?"=TRUE, "Can Write?"=FALSE, "Is Read?"=FALSE, "Is Write?"=FALSE, "Inactive Parent?"=FALSE, "Unwired?"=FALSE}, {"Label"="Has Caption", "Tag"="6332022.Has Caption", "Property Type"=enum."Scripting", "Indent"=0, "Can Read?"=TRUE, "Can Write?"=FALSE, "Is Read?"=FALSE, "Is Write?"=FALSE, "Inactive Parent?"=FALSE, "Unwired?"=FALSE}, {"Label"="Indicator", "Tag"="6332007.Indicator", "Property Type"=enum."Base", "Indent"=0, "Can Read?"=TRUE, "Can Write?"=TRUE, "Is Read?"=FALSE, "Is Write?"=FALSE, "Inactive Parent?"=FALSE, "Unwired?"=FALSE}, {"Label"="Invoke Nodes[]", "Tag"="633200c.Invoke Nodes[]", "Property Type"=enum."Scripting", "Indent"=0, "Can Read?"=TRUE, "Can Write?"=FALSE, "Is Read?"=FALSE, "Is Write?"=FALSE, "Inactive Parent?"=FALSE, "Unwired?"=FALSE}, {"Label"="Is On Connector Pane", "Tag"="6332020.Is On Connector Pane", "Property Type"=enum."Scripting", "Indent"=0, "Can Read?"=TRUE, "Can Write?"=FALSE, "Is Read?"=FALSE, "Is Write?"=FALSE, "Inactive Parent?"=FALSE, "Unwired?"=FALSE}, {"Label"="Is Stub?", "Tag"="633203b.Is Stub?", "Property Type"=enum."Private", "Indent"=0, "Can Read?"=TRUE, "Can Write?"=FALSE, "Is Read?"=FALSE, "Is Write?"=FALSE, "Inactive Parent?"=FALSE, "Unwired?"=FALSE}, {"Label"="Is Typedef?", "Tag"="633201a.Is Typedef?", "Property Type"=enum."Scripting", "Indent"=0, "Can Read?"=TRUE, "Can Write?"=FALSE, "Is Read?"=FALSE, "Is Write?"=FALSE, "Inactive Parent?"=FALSE, "Unwired?"=FALSE}, {"Label"="Key Focus", "Tag"="6332002.Key Focus", "Property Type"=enum."Base", "Indent"=0, "Can Read?"=TRUE, "Can Write?"=TRUE, "Is Read?"=FALSE, "Is Write?"=FALSE, "Inactive Parent?"=FALSE, "Unwired?"=FALSE}, {"Label"="Label", "Tag"="6332005.Label", "Property Type"=enum."Base", "Indent"=0, "Can Read?"=TRUE, "Can Write?"=FALSE, "Is Read?"=FALSE, "Is Write?"=FALSE, "Inactive Parent?"=FALSE, "Unwired?"=FALSE}, {"Label"="Latch Value", "Tag"="633201f.Latch Value", "Property Type"=enum."Private", "Indent"=0, "Can Read?"=TRUE, "Can Write?"=TRUE, "Is Read?"=FALSE, "Is Write?"=FALSE, "Inactive Parent?"=FALSE, "Unwired?"=FALSE}, {"Label"="Local Variables[]", "Tag"="633200a.Local Variables[]", "Property Type"=enum."Scripting", "Indent"=0, "Can Read?"=TRUE, "Can Write?"=FALSE, "Is Read?"=FALSE, "Is Write?"=FALSE, "Inactive Parent?"=FALSE, "Unwired?"=FALSE}, {"Label"="Owning Pane", "Tag"="633203e.Owning Pane", "Property Type"=enum."Base", "Indent"=0, "Can Read?"=TRUE, "Can Write?"=FALSE, "Is Read?"=FALSE, "Is Write?"=FALSE, "Inactive Parent?"=FALSE, "Unwired?"=FALSE}, {"Label"="Property Nodes[]", "Tag"="633200b.Property Nodes[]", "Property Type"=enum."Scripting", "Indent"=0, "Can Read?"=TRUE, "Can Write?"=FALSE, "Is Read?"=FALSE, "Is Write?"=FALSE, "Inactive Parent?"=FALSE, "Unwired?"=FALSE}, {"Label"="Skip When Tabbing", "Tag"="6332021.Skip When Tabbing", "Property Type"=enum."Base", "Indent"=0, "Can Read?"=TRUE, "Can Write?"=TRUE, "Is Read?"=FALSE, "Is Write?"=FALSE, "Inactive Parent?"=FALSE, "Unwired?"=FALSE}, {"Label"="Style ID", "Tag"="633203a.Style ID", "Property Type"=enum."Scripting", "Indent"=0, "Can Read?"=TRUE, "Can Write?"=FALSE, "Is Read?"=FALSE, "Is Write?"=FALSE, "Inactive Parent?"=FALSE, "Unwired?"=FALSE}, {"Label"="Synchronous Display", "Tag"="6332008.Synchronous Display", "Property Type"=enum."Base", "Indent"=0, "Can Read?"=TRUE, "Can Write?"=TRUE, "Is Read?"=FALSE, "Is Write?"=FALSE, "Inactive Parent?"=FALSE, "Unwired?"=FALSE}, {"Label"="Terminal", "Tag"="6332006.Terminal", "Property Type"=enum."Scripting", "Indent"=0, "Can Read?"=TRUE, "Can Write?"=FALSE, "Is Read?"=FALSE, "Is Write?"=FALSE, "Inactive Parent?"=FALSE, "Unwired?"=FALSE}, {"Label"="Tip Strip", "Tag"="6332014.Tip Strip", "Property Type"=enum."Base", "Indent"=0, "Can Read?"=TRUE, "Can Write?"=TRUE, "Is Read?"=FALSE, "Is Write?"=FALSE, "Inactive Parent?"=FALSE, "Unwired?"=FALSE}, {"Label"="Typedef", "Tag"="Typedef", "Property Type"=enum."Scripting", "Indent"=0, "Can Read?"=FALSE, "Can Write?"=FALSE, "Is Read?"=FALSE, "Is Write?"=FALSE, "Inactive Parent?"=TRUE, "Unwired?"=FALSE}, {"Label"="Path", "Tag"="633201b.Typedef:Path", "Property Type"=enum."Scripting", "Indent"=1, "Can Read?"=TRUE, "Can Write?"=FALSE, "Is Read?"=FALSE, "Is Write?"=FALSE, "Inactive Parent?"=FALSE, "Unwired?"=FALSE}, {"Label"="VI", "Tag"="6332025.Typedef:VI", "Property Type"=enum."Scripting", "Indent"=1, "Can Read?"=TRUE, "Can Write?"=FALSE, "Is Read?"=FALSE, "Is Write?"=FALSE, "Inactive Parent?"=FALSE, "Unwired?"=FALSE}, {"Label"="", "Tag"="", "Property Type"=enum."Base", "Indent"=0, "Can Read?"=FALSE, "Can Write?"=FALSE, "Is Read?"=FALSE, "Is Write?"=FALSE, "Inactive Parent?"=FALSE, "Unwired?"=FALSE}, {"Label"="", "Tag"="", "Property Type"=enum."Base", "Indent"=0, "Can Read?"=FALSE, "Can Write?"=FALSE, "Is Read?"=FALSE, "Is Write?"=FALSE, "Inactive Parent?"=FALSE, "Unwired?"=FALSE}, {"Label"="Value (Undoable)", "Tag"="6332041.Value (Undoable)", "Property Type"=enum."Scripting", "Indent"=0, "Can Read?"=FALSE, "Can Write?"=TRUE, "Is Read?"=FALSE, "Is Write?"=FALSE, "Inactive Parent?"=FALSE, "Unwired?"=FALSE}, {"Label"="Visible", "Tag"="6332000.Visible", "Property Type"=enum."Base", "Indent"=0, "Can Read?"=TRUE, "Can Write?"=TRUE, "Is Read?"=FALSE, "Is Write?"=FALSE, "Inactive Parent?"=FALSE, "Unwired?"=FALSE}, {"Label"="Wizard Data", "Tag"="6332019.Wizard Data", "Property Type"=enum."Private", "Indent"=0, "Can Read?"=TRUE, "Can Write?"=TRUE, "Is Read?"=FALSE, "Is Write?"=FALSE, "Inactive Parent?"=FALSE, "Unwired?"=FALSE}, {"Label"="XControl", "Tag"="XControl", "Property Type"=enum."Base", "Indent"=0, "Can Read?"=FALSE, "Can Write?"=FALSE, "Is Read?"=FALSE, "Is Write?"=FALSE, "Inactive Parent?"=TRUE, "Unwired?"=FALSE}, {"Label"="Container Bounds", "Tag"="6332037.XControl:Container Bounds", "Property Type"=enum."Base", "Indent"=1, "Can Read?"=TRUE, "Can Write?"=TRUE, "Is Read?"=FALSE, "Is Write?"=FALSE, "Inactive Parent?"=FALSE, "Unwired?"=FALSE}, {"Label"="XControl", "Tag"="XControl", "Property Type"=enum."Base", "Indent"=1, "Can Read?"=FALSE, "Can Write?"=FALSE, "Is Read?"=FALSE, "Is Write?"=FALSE, "Inactive Parent?"=TRUE, "Unwired?"=FALSE}, {"Label"="Container Bounds:Height", "Tag"="6332039.XControl:Container Bounds:Height", "Property Type"=enum."Base", "Indent"=2, "Can Read?"=TRUE, "Can Write?"=TRUE, "Is Read?"=FALSE, "Is Write?"=FALSE, "Inactive Parent?"=FALSE, "Unwired?"=FALSE}, {"Label"="Container Bounds:Width", "Tag"="6332038.XControl:Container Bounds:Width", "Property Type"=enum."Base", "Indent"=2, "Can Read?"=TRUE, "Can Write?"=TRUE, "Is Read?"=FALSE, "Is Write?"=FALSE, "Inactive Parent?"=FALSE, "Unwired?"=FALSE}, {"Label"="XControl", "Tag"="XControl", "Property Type"=enum."Base", "Indent"=0, "Can Read?"=FALSE, "Can Write?"=FALSE, "Is Read?"=FALSE, "Is Write?"=FALSE, "Inactive Parent?"=TRUE, "Unwired?"=FALSE}, {"Label"="Is XControl?", "Tag"="6332036.XControl:Is XControl?", "Property Type"=enum."Base", "Indent"=1, "Can Read?"=TRUE, "Can Write?"=FALSE, "Is Read?"=FALSE, "Is Write?"=FALSE, "Inactive Parent?"=FALSE, "Unwired?"=FALSE}, {"Label"="Adapt To Source", "Tag"="633b01e.Adapt To Source", "Property Type"=enum."Scripting", "Indent"=0, "Can Read?"=TRUE, "Can Write?"=TRUE, "Is Read?"=FALSE, "Is Write?"=FALSE, "Inactive Parent?"=FALSE, "Unwired?"=FALSE}, {"Label"="Data Entry Limits", "Tag"="633b004.Data Entry Limits", "Property Type"=enum."Base", "Indent"=0, "Can Read?"=TRUE, "Can Write?"=TRUE, "Is Read?"=FALSE, "Is Write?"=FALSE, "Inactive Parent?"=FALSE, "Unwired?"=FALSE}, {"Label"="Increment", "Tag"="633b007.Data Entry Limits:Increment", "Property Type"=enum."Base", "Indent"=1, "Can Read?"=TRUE, "Can Write?"=TRUE, "Is Read?"=FALSE, "Is Write?"=FALSE, "Inactive Parent?"=FALSE, "Unwired?"=FALSE}, {"Label"="Maximum", "Tag"="633b006.Data Entry Limits:Maximum", "Property Type"=enum."Base", "Indent"=1, "Can Read?"=TRUE, "Can Write?"=TRUE, "Is Read?"=FALSE, "Is Write?"=FALSE, "Inactive Parent?"=FALSE, "Unwired?"=FALSE}, {"Label"="Minimum", "Tag"="633b005.Data Entry Limits:Minimum", "Property Type"=enum."Base", "Indent"=1, "Can Read?"=TRUE, "Can Write?"=TRUE, "Is Read?"=FALSE, "Is Write?"=FALSE, "Inactive Parent?"=FALSE, "Unwired?"=FALSE}, {"Label"="Decrement Key Binding", "Tag"="633b011.Decrement Key Binding", "Property Type"=enum."Base", "Indent"=0, "Can Read?"=TRUE, "Can Write?"=TRUE, "Is Read?"=FALSE, "Is Write?"=FALSE, "Inactive Parent?"=FALSE, "Unwired?"=FALSE}, {"Label"="Fixed-Point Overflow Status Visible?", "Tag"="633b020.Fixed-Point Overflow Status Visible?", "Property Type"=enum."Private", "Indent"=0, "Can Read?"=TRUE, "Can Write?"=TRUE, "Is Read?"=FALSE, "Is Write?"=FALSE, "Inactive Parent?"=FALSE, "Unwired?"=FALSE}, {"Label"="Fixed-Point Representation", "Tag"="Fixed-Point Representation", "Property Type"=enum."Private", "Indent"=0, "Can Read?"=FALSE, "Can Write?"=FALSE, "Is Read?"=FALSE, "Is Write?"=FALSE, "Inactive Parent?"=TRUE, "Unwired?"=FALSE}, {"Label"="Actual", "Tag"="633b01a.Fixed-Point Representation:Actual", "Property Type"=enum."Private", "Indent"=1, "Can Read?"=TRUE, "Can Write?"=FALSE, "Is Read?"=FALSE, "Is Write?"=FALSE, "Inactive Parent?"=FALSE, "Unwired?"=FALSE}, {"Label"="Fixed-Point Representation", "Tag"="Fixed-Point Representation", "Property Type"=enum."Private", "Indent"=1, "Can Read?"=FALSE, "Can Write?"=FALSE, "Is Read?"=FALSE, "Is Write?"=FALSE, "Inactive Parent?"=TRUE, "Unwired?"=FALSE}, {"Label"="Actual:Delta", "Tag"="633b01d.Fixed-Point Representation:Actual:Delta", "Property Type"=enum."Private", "Indent"=2, "Can Read?"=TRUE, "Can Write?"=FALSE, "Is Read?"=FALSE, "Is Write?"=FALSE, "Inactive Parent?"=FALSE, "Unwired?"=FALSE}, {"Label"="Actual:Range Max", "Tag"="633b01c.Fixed-Point Representation:Actual:Range Max", "Property Type"=enum."Private", "Indent"=2, "Can Read?"=TRUE, "Can Write?"=FALSE, "Is Read?"=FALSE, "Is Write?"=FALSE, "Inactive Parent?"=FALSE, "Unwired?"=FALSE}, {"Label"="Actual:Range Min", "Tag"="633b01b.Fixed-Point Representation:Actual:Range Min", "Property Type"=enum."Private", "Indent"=2, "Can Read?"=TRUE, "Can Write?"=FALSE, "Is Read?"=FALSE, "Is Write?"=FALSE, "Inactive Parent?"=FALSE, "Unwired?"=FALSE}, {"Label"="Fixed-Point Representation", "Tag"="Fixed-Point Representation", "Property Type"=enum."Private", "Indent"=0, "Can Read?"=FALSE, "Can Write?"=FALSE, "Is Read?"=FALSE, "Is Write?"=FALSE, "Inactive Parent?"=TRUE, "Unwired?"=FALSE}, {"Label"="Bits", "Tag"="633b012.Fixed-Point Representation:Bits", "Property Type"=enum."Private", "Indent"=1, "Can Read?"=TRUE, "Can Write?"=TRUE, "Is Read?"=FALSE, "Is Write?"=FALSE, "Inactive Parent?"=FALSE, "Unwired?"=FALSE}, {"Label"="Fixed-Point Representation", "Tag"="Fixed-Point Representation", "Property Type"=enum."Private", "Indent"=1, "Can Read?"=FALSE, "Can Write?"=FALSE, "Is Read?"=FALSE, "Is Write?"=FALSE, "Inactive Parent?"=TRUE, "Unwired?"=FALSE}, {"Label"="Bits:Integer Word Length", "Tag"="633b015.Fixed-Point Representation:Bits:Integer Word Length", "Property Type"=enum."Private", "Indent"=2, "Can Read?"=TRUE, "Can Write?"=TRUE, "Is Read?"=FALSE, "Is Write?"=FALSE, "Inactive Parent?"=FALSE, "Unwired?"=FALSE}, {"Label"="Bits:Signed", "Tag"="633b013.Fixed-Point Representation:Bits:Signed", "Property Type"=enum."Private", "Indent"=2, "Can Read?"=TRUE, "Can Write?"=TRUE, "Is Read?"=FALSE, "Is Write?"=FALSE, "Inactive Parent?"=FALSE, "Unwired?"=FALSE}, {"Label"="Bits:Word Length", "Tag"="633b014.Fixed-Point Representation:Bits:Word Length", "Property Type"=enum."Private", "Indent"=2, "Can Read?"=TRUE, "Can Write?"=TRUE, "Is Read?"=FALSE, "Is Write?"=FALSE, "Inactive Parent?"=FALSE, "Unwired?"=FALSE}, {"Label"="Fixed-Point Representation", "Tag"="Fixed-Point Representation", "Property Type"=enum."Private", "Indent"=0, "Can Read?"=FALSE, "Can Write?"=FALSE, "Is Read?"=FALSE, "Is Write?"=FALSE, "Inactive Parent?"=TRUE, "Unwired?"=FALSE}, {"Label"="Desired", "Tag"="633b016.Fixed-Point Representation:Desired", "Property Type"=enum."Private", "Indent"=1, "Can Read?"=TRUE, "Can Write?"=TRUE, "Is Read?"=FALSE, "Is Write?"=FALSE, "Inactive Parent?"=FALSE, "Unwired?"=FALSE}, {"Label"="Fixed-Point Representation", "Tag"="Fixed-Point Representation", "Property Type"=enum."Private", "Indent"=1, "Can Read?"=FALSE, "Can Write?"=FALSE, "Is Read?"=FALSE, "Is Write?"=FALSE, "Inactive Parent?"=TRUE, "Unwired?"=FALSE}, {"Label"="Desired:Delta", "Tag"="633b019.Fixed-Point Representation:Desired:Delta", "Property Type"=enum."Private", "Indent"=2, "Can Read?"=TRUE, "Can Write?"=TRUE, "Is Read?"=FALSE, "Is Write?"=FALSE, "Inactive Parent?"=FALSE, "Unwired?"=FALSE}, {"Label"="Desired:Range Max", "Tag"="633b018.Fixed-Point Representation:Desired:Range Max", "Property Type"=enum."Private", "Indent"=2, "Can Read?"=TRUE, "Can Write?"=TRUE, "Is Read?"=FALSE, "Is Write?"=FALSE, "Inactive Parent?"=FALSE, "Unwired?"=FALSE}, {"Label"="Desired:Range Min", "Tag"="633b017.Fixed-Point Representation:Desired:Range Min", "Property Type"=enum."Private", "Indent"=2, "Can Read?"=TRUE, "Can Write?"=TRUE, "Is Read?"=FALSE, "Is Write?"=FALSE, "Inactive Parent?"=FALSE, "Unwired?"=FALSE}, {"Label"="Fixed-Point Representation", "Tag"="Fixed-Point Representation", "Property Type"=enum."Private", "Indent"=0, "Can Read?"=FALSE, "Can Write?"=FALSE, "Is Read?"=FALSE, "Is Write?"=FALSE, "Inactive Parent?"=TRUE, "Unwired?"=FALSE}, {"Label"="Include Overflow Status?", "Tag"="633b01f.Fixed-Point Representation:Include Overflow Status?", "Property Type"=enum."Private", "Indent"=1, "Can Read?"=TRUE, "Can Write?"=TRUE, "Is Read?"=FALSE, "Is Write?"=FALSE, "Inactive Parent?"=FALSE, "Unwired?"=FALSE}, {"Label"="Increment Key Binding", "Tag"="633b010.Increment Key Binding", "Property Type"=enum."Base", "Indent"=0, "Can Read?"=TRUE, "Can Write?"=TRUE, "Is Read?"=FALSE, "Is Write?"=FALSE, "Inactive Parent?"=FALSE, "Unwired?"=FALSE}, {"Label"="Representation", "Tag"="633b003.Representation", "Property Type"=enum."Scripting", "Indent"=0, "Can Read?"=TRUE, "Can Write?"=TRUE, "Is Read?"=FALSE, "Is Write?"=FALSE, "Inactive Parent?"=FALSE, "Unwired?"=FALSE}, {"Label"="Response to Value Outside Limits", "Tag"="633b00b.Response to Value Outside Limits", "Property Type"=enum."Base", "Indent"=0, "Can Read?"=TRUE, "Can Write?"=TRUE, "Is Read?"=FALSE, "Is Write?"=FALSE, "Inactive Parent?"=FALSE, "Unwired?"=FALSE}, {"Label"="Increment", "Tag"="633b00e.Response to Value Outside Limits:Increment", "Property Type"=enum."Base", "Indent"=1, "Can Read?"=TRUE, "Can Write?"=TRUE, "Is Read?"=FALSE, "Is Write?"=FALSE, "Inactive Parent?"=FALSE, "Unwired?"=FALSE}, {"Label"="Maximum", "Tag"="633b00c.Response to Value Outside Limits:Maximum", "Property Type"=enum."Base", "Indent"=1, "Can Read?"=TRUE, "Can Write?"=TRUE, "Is Read?"=FALSE, "Is Write?"=FALSE, "Inactive Parent?"=FALSE, "Unwired?"=FALSE}, {"Label"="Minimum", "Tag"="633b00d.Response to Value Outside Limits:Minimum", "Property Type"=enum."Base", "Indent"=1, "Can Read?"=TRUE, "Can Write?"=TRUE, "Is Read?"=FALSE, "Is Write?"=FALSE, "Inactive Parent?"=FALSE, "Unwired?"=FALSE}, {"Label"="Unit Label", "Tag"="633b00a.Unit Label", "Property Type"=enum."Base", "Indent"=0, "Can Read?"=TRUE, "Can Write?"=FALSE, "Is Read?"=FALSE, "Is Write?"=FALSE, "Inactive Parent?"=FALSE, "Unwired?"=FALSE}, {"Label"="Display Format", "Tag"="633bc06.Display Format", "Property Type"=enum."Base", "Indent"=0, "Can Read?"=TRUE, "Can Write?"=TRUE, "Is Read?"=FALSE, "Is Write?"=FALSE, "Inactive Parent?"=FALSE, "Unwired?"=FALSE}, {"Label"="Format", "Tag"="633bc07.Display Format:Format", "Property Type"=enum."Base", "Indent"=1, "Can Read?"=TRUE, "Can Write?"=TRUE, "Is Read?"=FALSE, "Is Write?"=FALSE, "Inactive Parent?"=FALSE, "Unwired?"=FALSE}, {"Label"="Precision", "Tag"="633bc08.Display Format:Precision", "Property Type"=enum."Base", "Indent"=1, "Can Read?"=TRUE, "Can Write?"=TRUE, "Is Read?"=FALSE, "Is Write?"=FALSE, "Inactive Parent?"=FALSE, "Unwired?"=FALSE}, {"Label"="Format String", "Tag"="633bc05.Format String", "Property Type"=enum."Base", "Indent"=0, "Can Read?"=TRUE, "Can Write?"=TRUE, "Is Read?"=FALSE, "Is Write?"=FALSE, "Inactive Parent?"=FALSE, "Unwired?"=FALSE}, {"Label"="Hide Text", "Tag"="633bc09.Hide Text", "Property Type"=enum."Private", "Indent"=0, "Can Read?"=TRUE, "Can Write?"=TRUE, "Is Read?"=FALSE, "Is Write?"=FALSE, "Inactive Parent?"=FALSE, "Unwired?"=FALSE}, {"Label"="Increment/Decrement Visible?", "Tag"="633bc04.Increment/Decrement Visible?", "Property Type"=enum."Base", "Indent"=0, "Can Read?"=TRUE, "Can Write?"=TRUE, "Is Read?"=FALSE, "Is Write?"=FALSE, "Inactive Parent?"=FALSE, "Unwired?"=FALSE}, {"Label"="Numeric Text", "Tag"="633bc03.Numeric Text", "Property Type"=enum."Base", "Indent"=0, "Can Read?"=TRUE, "Can Write?"=FALSE, "Is Read?"=FALSE, "Is Write?"=FALSE, "Inactive Parent?"=FALSE, "Unwired?"=FALSE}, {"Label"="Radix Visible?", "Tag"="633bc02.Radix Visible?", "Property Type"=enum."Base", "Indent"=0, "Can Read?"=TRUE, "Can Write?"=TRUE, "Is Read?"=FALSE, "Is Write?"=FALSE, "Inactive Parent?"=FALSE, "Unwired?"=FALSE}, {"Label"="Text Width", "Tag"="633bc01.Text Width", "Property Type"=enum."Base", "Indent"=0, "Can Read?"=TRUE, "Can Write?"=TRUE, "Is Read?"=FALSE, "Is Write?"=FALSE, "Inactive Parent?"=FALSE, "Unwired?"=FALSE}] ("Properties for Tree Out"), s=w56, f=w47) -> (s? t:f=w53:T5)
      n17 = call <userlib>:"Current VIs Reference__ogtk.vi"() -> ("Current VI's reference"=w49:refnum<vi>)  [unwired: 5 in]
      n18 = call "Property Tree_Populate Trees.vi"("Close Items"=w46, "VI Ref"=w49, "Filter"="", "Action"=w52, "Error In"=w38, "Tree Refs"=w51, "Show"=w50, "Properties for Tree In"=w53) -> ("error out"=w55:errorcluster)  [unwired: 3 in]
      n19 = call "Tree_Setup for dialog.vi"("Action"=w52, "error in"=w55, "Tree Ref"=w51) -> ("error out"=w45:errorcluster)  [unwired: 7 in, 1 out]
      n20 = call "Dialog Window Setup.vi"("Action"=enum16{"Pre-Populate", "Post-Populate"}."Post-Populate", "error in"=w45, "Dialog VI Ref In [Parent]"=w44) -> ("error out"=w40:errorcluster, "Dialog VI Ref Out"=w43:refnum<vi>)  [unwired: 7 in]
      n21 = control-ref of="Filter"() -> (w41:refnum<vi>)
      n22 = call "Dialog_Setup Filter String.vi"("Action"=w39, "error in"=w40, "Filter String Ref"=w41) -> ("error out"=w37:errorcluster)  [unwired: 7 in, 1 out]
    }
  }
  n23 = call <vilib>:"Simple Error Handler.vi"("error in (no error)"=w2) -> ("error out"=→"Error Out":errorcluster)  [unwired: 4 in, 4 out]
  n24 = while {
    tunnel: w13 -> [w61]
    tunnel: [w60] -> w19
    tunnel: [w59] -> w16
    tunnel: w17 -> [w59]
    tunnel: w9 -> [w58]
    tunnel: w7 -> [w57]
    stop <- w62 stop-if-true
    n25 = event shown="[0] \"Done\": Value Change" {
      selector: _ -> [_ _ _ _ _ _ _ _]
      dyn-events: _ -> [_ _ _ _ _ _ _ _]
      timeout: _ -> [_ _ _ _ _ _ _ _]
      tunnel: [w64 _ _ _ w101 _ w122 w127] -> w62
      tunnel: w61 -> [_ _ w72 w86 w105 w109 _ _]
      tunnel: [TRUE _ _ _ w101 _ _ _] -> w60
      tunnel: w58 -> [_ _ w80 _ _ _ _ _]
      tunnel: w57 -> [_ _ w73 _ _ _ _ _]
      event Value Change {
        n26 = event-data() -> ("NewVal"=w64:T2)  [unwired: 1 in]
      }
      event Key Down? {
        n27 = event-data() -> ("Char"=w66:i16)  [unwired: 1 in]
        n28 = case shown="9" w66 {
          tunnel: [_ TRUE ("Discard?")] -> w65
          frame 0, Default {
          }
          frame 9 {
            # "Tab"
            n29 = control-ref of="Filter"() -> (w67:refnum<vi>)
            n30 = call "Filter_Set focus.vi"("Fillter String Ref"=w67) -> ()  [unwired: 10 in, 1 out]
          }
        }
        n31 = event-data("Discard?"=w65) -> ()  [unwired: 1 in, 1 out]
      }
      event "Property Display", "Filter": Value Change {
        w69 = FALSE  # Close Items
        n32 = event-data() -> ()  [unwired: 1 in, 1 out]
        n33 = Equal?(x="Filter..." ("Default Value"), y="Filter") -> (x = y?=w79:bool)
        n34 = Select(t="", s=w79, f="Filter") -> (s? t:f=w75:string)
        n35 = call <userlib>:"Current VIs Reference__ogtk.vi"() -> ("Current VI's reference"=w74:refnum<vi>)  [unwired: 5 in]
        n36 = call "Property Tree_Populate Trees.vi"("Close Items"=w69, "VI Ref"=w74, "Filter"=w75, "Action"=w80, "Tree Refs"=w72, "Show"="Property Display", "Properties for Tree In"=w73) -> ()  [unwired: 4 in, 1 out]
        n37 = call "INI_Dialog display options.vi"("File Action"=enum16{"Read", "Write"}."Write", "Display Options"="Property Display") -> ()  [unwired: 9 in, 1 out]
      }
      event "Filter": Key Down? {
        n38 = event-data() -> ("ScanCode"=w85:i16, "VKey"=w84:T7)  [unwired: 1 in]
        n39 = control-ref of="Done"() -> (w81:refnum<vi>)
        n40 = Index Array(array=w86) -> (element=w83:refnum<vi>)  [unwired: 1 in]
        n41 = case shown="Default" w84 {
          tunnel: [w89 TRUE TRUE] -> w82
          tunnel: w83 -> [w90 w95 w99]
          tunnel: w85 -> [w88 _ _]
          tunnel: w81 -> [w87 _ _]
          frame Default {
            n42 = case shown="15" w88 {
              tunnel: w90 -> [_ w94]
              tunnel: [_ TRUE] -> w89
              tunnel: w87 -> [_ w91]
              frame 0, Default {
              }
              frame 15 {
                # "TAB"
                n43 = call "Tree_Select first or last item.vi"("Select Item"=enum16{"First", "Last"}."First", "Done Ref"=w91, "Tree Ref"=w94) -> ()  [unwired: 7 in, 2 out]
              }
            }
          }
          frame "Down" {
            n44 = call "Class Tree_Select first or last item.vi"("Select Item"=enum16{"First", "Last"}."First", "Tree Ref"=w95) -> ()  [unwired: 9 in, 1 out]
          }
          frame "Up" {
            n45 = call "Class Tree_Select first or last item.vi"("Select Item"=enum16{"First", "Last"}."Last", "Tree Ref"=w99) -> ()  [unwired: 9 in, 1 out]
          }
        }
        n46 = event-data("Discard?"=w82) -> ()  [unwired: 1 in, 1 out]
      }
      event "Tree": Double Click {
        # "double click on disbale item ignored, else end dialog and read off selected item"
        n47 = event-data() -> ("Tag"=w103:string)  [unwired: 1 in]
        n48 = Index Array(array=w105) -> (element=w104:refnum<vi>)  [unwired: 1 in]
        n49 = property class="Tree"(reference=w104, "Active Item Tag"=w103) -> ("Disabled?"=w102:bool)  [unwired: 1 in, 2 out]
        n50 = Not(x=w102) -> (.not. x?=w101:bool)
      }
      event "Tree": Key Down? {
        # "Tabbing off the wasn't working so I added this"
        n51 = event-data() -> ("VKey"=w110:T7, "ScanCode"=w106:i16)  [unwired: 1 in]
        n52 = Index Array(array=w109) -> (element=w108:refnum<vi>)  [unwired: 1 in]
        n53 = case shown="Default" w110 {
          tunnel: [w112 w116 w120] -> w107
          tunnel: w108 -> [_ w118 w121]
          tunnel: w106 -> [w111 _ _]
          frame Default {
            n54 = case shown="15" w111 {
              tunnel: [_ TRUE ("discard")] -> w112
              frame 0, Default {
              }
              frame 15 {
                # "TAB"
                n55 = control-ref of="Done"() -> (w115:refnum<vi>)
                n56 = property class="Bool"(reference=w115, "Key Focus"=TRUE) -> ()  [unwired: 1 in, 2 out]
              }
            }
          }
          frame "Up" {
            n57 = call "Class Tree_Arrow Control.vi"("Direction"=enum16{"Down", "Up"}."Up", "Tree ref"=w118) -> ("discard"=w116:bool)  [unwired: 8 in, 1 out]
          }
          frame "Down" {
            n58 = call "Class Tree_Arrow Control.vi"("Direction"=enum16{"Down", "Up"}."Down", "Tree ref"=w121) -> ("discard"=w120:bool)  [unwired: 8 in, 1 out]
          }
        }
        n59 = event-data("Discard?"=w107) -> ()  [unwired: 1 in, 1 out]
      }
      event Key Down? {
        # "Quit on escape"
        n60 = event-data() -> ("VKey"=w123:T7)  [unwired: 1 in, 1 out]
        n61 = case shown="\"Escape\"" w123 {
          tunnel: [FALSE TRUE] -> w122
          frame Default {
          }
          frame "Escape" {
            # "Close window and return no value on esc"
          }
        }
        n62 = event-data("Discard?"=w122) -> ()  [unwired: 1 in, 1 out]
      }
      event Panel Close? {
        w127 = TRUE
        # "close and return no value on panel close"
        n63 = event-data() -> ()  [unwired: 1 in, 1 out]
        n64 = call "Is VI Running Top Level.vi"() -> ("Top Level?"=w126:bool)  [unwired: 5 in]
        n65 = case shown="False" w126 {
          frame False {
            n66 = invoke class="VI" method="FP.Close"() -> ()  [unwired: 3 in, 3 out]
          }
          frame True {
          }
        }
        n67 = event-data("Discard?"=w127) -> ()  [unwired: 1 in, 1 out]
      }
    }
  }
  n68 = call "Is VI Running Top Level.vi"() -> ("Top Level?"=w14:bool)  [unwired: 5 in]
  n69 = case shown="True" w19 {
    tunnel: [T3 [] ("Property Array Out") w131] -> w8
    tunnel: [_ "Placement"] -> w5
    frame False {
    }
    frame True {
      n70 = for {
        tunnel: "Tree" -> [w133] mode=indexing
        tunnel: [w132] -> w131 mode=indexing
        n71 = Bundle(cluster=T8 {"Tag"="", "Read"=FALSE, "Write"=FALSE, "New"=FALSE} ("Property Tree Element Value"), "Tag"=w133) -> (w132:T8)  [unwired: 3 in]
      }
    }
  }
  "Method Array Out" <- w8
  "Placement Out" <- w5
  n72 = case shown="True" w14 {
    tunnel: w16 -> [w136 w137]
    tunnel: [w135 w137] -> w15
    frame False {
      n73 = invoke class="VI" method="FP.Close"(reference=w136) -> (reference out=w135:refnum<vi>)  [unwired: 2 in, 2 out]
    }
    frame True {
    }
  }
  n74 = call "FP splitter mode handler.vi"("Mode"=enum16{"Run", "Development"}."Development", "VI Ref In"=w15) -> ()  [unwired: 8 in, 2 out]
